vi "Version_4.9_8_on-chip_valves_for25ulSyringe_withModfied_Plunging.vi"() -> ()   [LabVIEW 2020] (continued)
                            n7037 = call "PortChanger (SubVI).vi"("Port Number"=w7491, "VISA Refnum in"=w7492) -> ()  [unwired: 10 in]
                          }
                          frame #1 {
                            n7038 = local read "VISA Refnum in\nfor Pump"() -> (w7493:refnum<visa-resource-name>)
                            n7039 = call "ProcessCompletionWaiter (SubVI).vi"("VISA Refnum in"=w7493) -> ()  [unwired: 11 in]
                          }
                          frame #2 {
                            n7040 = local read "Buffer-A2 PickUp \nFlow Rate (ul/min)"() -> (w7496:dbl)
                            n7041 = local read "Buffer-A2 Pumping\nResolution"() -> (w7495:T2)
                            n7042 = local read "VISA Refnum in\nfor Pump"() -> (w7498:refnum<visa-resource-name>)
                            n7043 = local read "Reminder of the \nVolume to be \nPumped"() -> (w7494:dbl)
                            n7044 = local read "Volume of Syringe"() -> (w7497:dbl)
                            n7045 = call "RPickUp(SubVI).vi"("Volume to be picked up"=w7494, "Volume of Syringe"=w7497, "Resolution of PickUP"=w7495, "PickUp Flow Rate (ul/min)"=w7496, "VISA Refnum in"=w7498) -> ()  [unwired: 6 in, 1 out]
                          }
                          frame #3 {
                            n7046 = local read "Stopper that ends \nthe main loops"() -> (w7499:bool)
                            n7047 = local read "VISA Refnum in\nfor Pump"() -> (w7500:refnum<visa-resource-name>)
                            n7048 = case shown="True" w7499 {
                              frame False {
                              }
                              frame True {
                                n7049 = local read "VISA Refnum in\nfor Pump"() -> (w7501:refnum<visa-resource-name>)
                                n7050 = call "HardStopCurrentProcess (SubVI).vi"("VISA Refnum in"=w7501) -> ()  [unwired: 11 in]
                              }
                            }
                            n7051 = call "ProcessCompletionWaiter (SubVI).vi"("VISA Refnum in"=w7500) -> ()  [unwired: 11 in]
                          }
                          frame #4 {
                            # "Reads the initial Plunger Position for computing the volume dispensed"
                            n7052 = local read "VISA Refnum in\nfor Pump"() -> (w7503:refnum<visa-resource-name>)
                            n7053 = call "AbsolutePlungerPosition (SubVI).vi"("VISA Refnum in"=w7503) -> ("Plunger Position"=w7502:i32)  [unwired: 10 in]
                            n7054 = local write "Initial Plunger Position"(w7502) -> ()
                          }
                          frame #5 {
                            # "Switch to Port-2"
                            # "Port-2 of the pump is conncted to column-1 of chip"
                            n7055 = local read "VISA Refnum in\nfor Pump"() -> (w7505:refnum<visa-resource-name>)
                            n7056 = call "PortChanger (SubVI).vi"("Port Number"="2", "VISA Refnum in"=w7505) -> ()  [unwired: 10 in]
                          }
                          frame #6 {
                            n7057 = local read "Stopper that ends \nthe main loops"() -> (w7506:bool)
                            n7058 = local read "VISA Refnum in\nfor Pump"() -> (w7507:refnum<visa-resource-name>)
                            n7059 = case shown="True" w7506 {
                              frame False {
                              }
                              frame True {
                                n7060 = local read "VISA Refnum in\nfor Pump"() -> (w7508:refnum<visa-resource-name>)
                                n7061 = call "HardStopCurrentProcess (SubVI).vi"("VISA Refnum in"=w7508) -> ()  [unwired: 11 in]
                              }
                            }
                            n7062 = call "ProcessCompletionWaiter (SubVI).vi"("VISA Refnum in"=w7507) -> ()  [unwired: 11 in]
                          }
                          frame #7 {
                            # "Keeps the AMF valve after column-1 open and valve after column-2 closed"
                            n7063 = local read "Buffer-A2 Dispense\nFlow Rate (ul/min)"() -> (w7521:dbl)
                            n7064 = local read "Buffer-A2 Pumping\nResolution"() -> (w7520:T2)
                            n7065 = local read "VISA Refnum in\nfor Pump"() -> (w7523:refnum<visa-resource-name>)
                            n7066 = local write "Pause Data Collection"(FALSE ("Pause Data Collection")) -> ()
                            n7067 = local write "Valve V3 Open"(FALSE ("Valve V3 Open")) -> ()
                            n7068 = local write "Valve V4 Open"(FALSE ("Valve V4 Open")) -> ()
                            n7069 = local write "Valve V1 Open"(TRUE ("Valve V1 Open")) -> ()
                            n7070 = local write "Valve V2 Open"(TRUE ("Valve V2 Open")) -> ()
                            n7071 = local read "Volume of Syringe"() -> (w7522:dbl)
                            n7072 = call "GoToAbsolutePosition(SubVI).vi"("Absolute Volume Position in Syringe (in ul)"=0.0 ("Volume to be Dispensed"), "Volume of Syringe"=w7522, "Resolution of Pumping"=w7520, "Flow Rate (ul/min)"=w7521, "VISA Refnum in"=w7523) -> ()  [unwired: 6 in, 1 out]
                            n7073 = local write "External Valve \nOpen"(TRUE ("External Valve \nOpen")) -> ()
                            n7074 = local write "Valve V5 Open"(FALSE ("Valve V5 Open")) -> ()
                            n7075 = local write "Valve V8 Open"(FALSE ("Valve V8 Open")) -> ()
                            n7076 = local write "Valve V6 Open"(FALSE ("Valve V6 Open")) -> ()
                            n7077 = local write "Valve V7 Open"(FALSE ("Valve V7 Open")) -> ()
                          }
                          frame #8 {
                            n7078 = local read "Initial Plunger Position"() -> (w7526:dbl)
                            n7079 = local read "Buffer-A2 Pumping\nResolution"() -> (w7525:T2)
                            n7080 = local read "VISA Refnum in\nfor Pump"() -> (w7527:refnum<visa-resource-name>)
                            n7081 = local read "Volume of Syringe"() -> (w7524:dbl)
                            n7082 = while {
                              tunnel: w7526 -> [w7533]
                              tunnel: w7527 -> [w7532]
                              tunnel: w7525 -> [w7531]
                              tunnel: w7524 -> [w7530]
                              stop <- w7528 stop-if-true
                              n7083 = Wait (ms)(milliseconds to wait=u32 100) -> ()  [unwired: 1 out]
                              n7084 = stacked-sequence {
                                tunnel: w7533 -> [w7539 _]
                                tunnel: w7532 -> [w7538 w7559]
                                tunnel: w7531 -> [w7537 _]
                                tunnel: w7530 -> [w7536 _]
                                tunnel: [_ w7556] -> w7528
                                frame #0 {
                                n7085 = call "AbsolutePlungerPosition (SubVI).vi"("VISA Refnum in"=w7538) -> ("Plunger Position"=w7535:i32)  [unwired: 10 in]
                                n7086 = case shown="\"Standard Pumping\", Default" w7537 {
                                tunnel: w7539 -> [w7544 w7553]
                                tunnel: w7535 -> [w7545 w7552]
                                tunnel: [w7543 w7550] -> w7534
                                tunnel: w7536 -> [w7542 w7551]
                                frame "Standard Pumping", Default {
                                n7087 = Subtract(x=w7544, y=w7545) -> (x-y=w7541:dbl)
                                n7088 = Absolute Value(x=w7541) -> (abs(x)=w7540:dbl)
                                n7089 = Multiply(x=w7540, y=w7542) -> (x*y=w7547:dbl)
                                n7090 = Divide(x=w7547, y=3000.0) -> (x/y=w7543:dbl)
                                }
                                frame "High Resolution Pumping" {
                                n7091 = Subtract(x=w7553, y=w7552) -> (x-y=w7549:dbl)
                                n7092 = Absolute Value(x=w7549) -> (abs(x)=w7548:dbl)
                                n7093 = Multiply(x=w7548, y=w7551) -> (x*y=w7555:dbl)
                                n7094 = Divide(x=w7555, y=24000.0) -> (x/y=w7550:dbl)
                                }
                                }
                                n7095 = local write "Volume being Injected \nin this process"(w7534) -> ()
                                }
                                frame #1 {
                                n7096 = local read "Stop for End of \nExperiment \nand Data Writing"() -> (w7558:bool)
                                n7097 = call "LSPOneStatus (SubVI).vi"("VISA Refnum in"=w7559) -> ("read buffer"=w7561:string)  [unwired: 10 in]
                                n7098 = call <vilib>:"Trim Whitespace.vi"("string"=w7561) -> ("trimmed string"=w7560:string)  [unwired: 1 in]
                                n7099 = Equal?(x=w7560, y="/0`\u0003") -> (x = y?=w7557:bool)
                                n7100 = Or(x=w7557, y=w7558) -> (x .or. y?=w7556:bool)
                                }
                              }
                            }
                          }
                          frame #9 {
                            n7101 = local read "Stop for End of \nExperiment \nand Data Writing"() -> (w7563:bool)
                            n7102 = local write "Pause Data Collection"(TRUE ("Pause Data Collection")) -> ()
                            n7103 = local write "Valve V3 Open"(FALSE ("Valve V3 Open")) -> ()
                            n7104 = local write "Valve V2 Open"(FALSE ("Valve V2 Open")) -> ()
                            n7105 = local write "Valve V4 Open"(FALSE ("Valve V4 Open")) -> ()
                            n7106 = local write "Start the Process"(FALSE) -> ()
                            n7107 = local write "Valve V1 Open"(FALSE ("Valve V1 Open")) -> ()
                            n7108 = case shown="True" w7563 {
                              frame False {
                              }
                              frame True {
                                n7109 = local read "VISA Refnum in\nfor Pump"() -> (w7574:refnum<visa-resource-name>)
                                n7110 = call "HardStopCurrentProcess (SubVI).vi"("VISA Refnum in"=w7574) -> ()  [unwired: 11 in]
                              }
                            }
                            n7111 = Wait (ms)(milliseconds to wait=u32 500) -> ()  [unwired: 1 out]
                            n7112 = local write "Valve V5 Open"(FALSE ("Valve V5 Open")) -> ()
                            n7113 = local write "Valve V6 Open"(FALSE ("Valve V6 Open")) -> ()
                            n7114 = local write "Valve V7 Open"(FALSE ("Valve V7 Open")) -> ()
                          }
                          frame #10 {
                            n7115 = local write "Volume being Injected \nin this process"(0.0 ("Volume being Injected \nin this process")) -> ()
                          }
                        }
                      }
                    }
                  }
                }
              }
              frame True {
                n7116 = local write "Pause Data Collection"(FALSE ("Pause Data Collection")) -> ()
              }
            }
          }
          frame "Inject Buffer B, Column 1 with 4 SOD Valves" {
            n7117 = local read "Stopper that ends \nthe main loops"() -> (w7577:bool)
            n7118 = case shown="False" w7577 {
              frame False {
                n7119 = local read "Start the Process"() -> (w7578:bool)
                n7120 = case shown="True" w7578 {
                  frame False {
                    n7121 = local read "Stopper that ends \nthe main loops"() -> (w7580:bool)
                    n7122 = local read "Start the Process"() -> (w7579:bool)
                    n7123 = Or(x=w7580, y=w7579) -> (x .or. y?=w7581:bool)
                    n7124 = case shown="False" w7581 {
                      frame False {
                        n7125 = while {
                          stop <- w7584 stop-if-true
                          n7126 = local read "Stop for End of \nExperiment \nand Data Writing"() -> (w7583:bool)
                          n7127 = local read "Stopper that ends \nthe main loops"() -> (w7586:bool)
                          n7128 = local read "Start the Process"() -> (w7585:bool)
                          n7129 = Wait (ms)(milliseconds to wait=u32 10) -> ()  [unwired: 1 out]
                          n7130 = Or(x=w7586, y=w7585) -> (x .or. y?=w7584:bool)
                          n7131 = local write "Stopper that ends \nthe main loops"(w7583) -> ()
                        }
                        n7132 = One Button Dialog(message="Please Select the Process and Press 'Start the Process' Button") -> ()  [unwired: 1 in, 1 out]
                      }
                      frame True {
                      }
                    }
                  }
                  frame True {
                    n7133 = stacked-sequence {
                      frame #0 {
                        n7134 = local read "Apparent Volume\nof Syringe"() -> (w7590:dbl)
                        n7135 = local read "Buffer-B Volume \nto be  Pumped"() -> (w7591:dbl)
                        n7136 = Quotient & Remainder(x=w7591, y=w7590) -> (x-y*floor(x/y)=w7588:dbl, floor(x/y)=w7589:dbl)
                        n7137 = for {
                          N: w7589 -> [_]
                          n7138 = stacked-sequence {
                            frame #0 {
                              # "Switch to Port-7"
                              # "Port-7 of pump is connected to Buffer-B"
                              n7139 = local read "VISA Refnum in\nfor Pump"() -> (w7593:refnum<visa-resource-name>)
                              n7140 = local read "Port for \nB-Elution"() -> (w7592:string)
                              n7141 = call "PortChanger (SubVI).vi"("Port Number"=w7592, "VISA Refnum in"=w7593) -> ()  [unwired: 10 in]
                            }
                            frame #1 {
                              n7142 = local read "VISA Refnum in\nfor Pump"() -> (w7594:refnum<visa-resource-name>)
                              n7143 = call "ProcessCompletionWaiter (SubVI).vi"("VISA Refnum in"=w7594) -> ()  [unwired: 11 in]
                            }
                            frame #2 {
                              n7144 = local read "Buffer-B PickUp \nFlow Rate (ul/min)"() -> (w7597:dbl)
                              n7145 = local read "Buffer-B Pumping\nResolution"() -> (w7596:T2)
                              n7146 = local read "VISA Refnum in\nfor Pump"() -> (w7599:refnum<visa-resource-name>)
                              n7147 = local read "Apparent Volume\nof Syringe"() -> (w7595:dbl)
                              n7148 = local read "Volume of Syringe"() -> (w7598:dbl)
                              n7149 = call "RPickUp(SubVI).vi"("Volume to be picked up"=w7595, "Volume of Syringe"=w7598, "Resolution of PickUP"=w7596, "PickUp Flow Rate (ul/min)"=w7597, "VISA Refnum in"=w7599) -> ()  [unwired: 6 in, 1 out]
                            }
                            frame #3 {
                              n7150 = local read "Stopper that ends \nthe main loops"() -> (w7600:bool)
                              n7151 = local read "VISA Refnum in\nfor Pump"() -> (w7601:refnum<visa-resource-name>)
                              n7152 = case shown="True" w7600 {
                                frame False {
                                }
                                frame True {
                                n7153 = local read "VISA Refnum in\nfor Pump"() -> (w7602:refnum<visa-resource-name>)
                                n7154 = call "HardStopCurrentProcess (SubVI).vi"("VISA Refnum in"=w7602) -> ()  [unwired: 11 in]
                                }
                              }
                              n7155 = call "ProcessCompletionWaiter (SubVI).vi"("VISA Refnum in"=w7601) -> ()  [unwired: 11 in]
                            }
                            frame #4 {
                              # "Reads the initial Plunger Position for computing the volume dispensed"
                              n7156 = local read "VISA Refnum in\nfor Pump"() -> (w7604:refnum<visa-resource-name>)
                              n7157 = call "AbsolutePlungerPosition (SubVI).vi"("VISA Refnum in"=w7604) -> ("Plunger Position"=w7603:i32)  [unwired: 10 in]
                              n7158 = local write "Initial Plunger Position"(w7603) -> ()
                            }
                            frame #5 {
                              # "Switch to Port-8"
                              # "Port-8 of the pump is conncted to column-1 of chip"
                              n7159 = local read "VISA Refnum in\nfor Pump"() -> (w7606:refnum<visa-resource-name>)
                              n7160 = call "PortChanger (SubVI).vi"("Port Number"="8", "VISA Refnum in"=w7606) -> ()  [unwired: 10 in]
                            }
                            frame #6 {
                              n7161 = local read "Stopper that ends \nthe main loops"() -> (w7607:bool)
                              n7162 = local read "VISA Refnum in\nfor Pump"() -> (w7608:refnum<visa-resource-name>)
                              n7163 = case shown="True" w7607 {
                                frame False {
                                }
                                frame True {
                                n7164 = local read "VISA Refnum in\nfor Pump"() -> (w7609:refnum<visa-resource-name>)
                                n7165 = call "HardStopCurrentProcess (SubVI).vi"("VISA Refnum in"=w7609) -> ()  [unwired: 11 in]
                                }
                              }
                              n7166 = call "ProcessCompletionWaiter (SubVI).vi"("VISA Refnum in"=w7608) -> ()  [unwired: 11 in]
                            }
                            frame #7 {
                              # "Keeps the AMF valve after column-1 open and valve after column-2 closed"
                              n7167 = local read "Buffer-B Dispense\nFlow Rate (ul/min)"() -> (w7622:dbl)
                              n7168 = local read "Buffer-B Pumping\nResolution"() -> (w7621:T2)
                              n7169 = local read "VISA Refnum in\nfor Pump"() -> (w7624:refnum<visa-resource-name>)
                              n7170 = local write "Pause Data Collection"(FALSE ("Pause Data Collection")) -> ()
                              n7171 = local write "Valve V1 Open"(TRUE ("Valve V1 Open")) -> ()
                              n7172 = local write "Valve V3 Open"(FALSE ("Valve V3 Open")) -> ()
                              n7173 = local write "Valve V2 Open"(TRUE ("Valve V2 Open")) -> ()
                              n7174 = local write "Valve V4 Open"(FALSE ("Valve V4 Open")) -> ()
                              n7175 = local read "Volume of Syringe"() -> (w7623:dbl)
                              n7176 = call "GoToAbsolutePosition(SubVI).vi"("Absolute Volume Position in Syringe (in ul)"=0.0 ("Volume to be Dispensed"), "Volume of Syringe"=w7623, "Resolution of Pumping"=w7621, "Flow Rate (ul/min)"=w7622, "VISA Refnum in"=w7624) -> ()  [unwired: 6 in, 1 out]
                              n7177 = local write "External Valve \nOpen"(TRUE ("External Valve \nOpen")) -> ()
                              n7178 = local write "Valve V8 Open"(FALSE ("Valve V8 Open")) -> ()
                              n7179 = local write "Valve V6 Open"(FALSE ("Valve V6 Open")) -> ()
                              n7180 = local write "Valve V7 Open"(FALSE ("Valve V7 Open")) -> ()
                              n7181 = local write "Valve V5 Open"(FALSE ("Valve V5 Open")) -> ()
                            }
                            frame #8 {
                              n7182 = local read "Initial Plunger Position"() -> (w7627:dbl)
                              n7183 = local read "Buffer-B Pumping\nResolution"() -> (w7626:T2)
                              n7184 = local read "VISA Refnum in\nfor Pump"() -> (w7628:refnum<visa-resource-name>)
                              n7185 = local read "Volume of Syringe"() -> (w7625:dbl)
                              n7186 = while {
                                tunnel: w7627 -> [w7634]
                                tunnel: w7628 -> [w7633]
                                tunnel: w7626 -> [w7632]
                                tunnel: w7625 -> [w7631]
                                stop <- w7629 stop-if-true
                                n7187 = Wait (ms)(milliseconds to wait=u32 100) -> ()  [unwired: 1 out]
                                n7188 = stacked-sequence {
                                tunnel: w7634 -> [w7640 _]
                                tunnel: w7633 -> [w7639 w7660]
                                tunnel: w7632 -> [w7638 _]
                                tunnel: w7631 -> [w7637 _]
                                tunnel: [_ w7657] -> w7629
                                frame #0 {
                                n7189 = call "AbsolutePlungerPosition (SubVI).vi"("VISA Refnum in"=w7639) -> ("Plunger Position"=w7636:i32)  [unwired: 10 in]
                                n7190 = case shown="\"Standard Pumping\", Default" w7638 {
                                tunnel: w7640 -> [w7645 w7654]
                                tunnel: w7636 -> [w7646 w7653]
                                tunnel: [w7644 w7651] -> w7635
                                tunnel: w7637 -> [w7643 w7652]
                                frame "Standard Pumping", Default {
                                n7191 = Subtract(x=w7645, y=w7646) -> (x-y=w7642:dbl)
                                n7192 = Absolute Value(x=w7642) -> (abs(x)=w7641:dbl)
                                n7193 = Multiply(x=w7641, y=w7643) -> (x*y=w7648:dbl)
                                n7194 = Divide(x=w7648, y=3000.0) -> (x/y=w7644:dbl)
                                }
                                frame "High Resolution Pumping" {
                                n7195 = Subtract(x=w7654, y=w7653) -> (x-y=w7650:dbl)
                                n7196 = Absolute Value(x=w7650) -> (abs(x)=w7649:dbl)
                                n7197 = Multiply(x=w7649, y=w7652) -> (x*y=w7656:dbl)
                                n7198 = Divide(x=w7656, y=24000.0) -> (x/y=w7651:dbl)
                                }
                                }
                                n7199 = local write "Volume being Injected \nin this process"(w7635) -> ()
                                }
                                frame #1 {
                                n7200 = call "LSPOneStatus (SubVI).vi"("VISA Refnum in"=w7660) -> ("read buffer"=w7662:string)  [unwired: 10 in]
                                n7201 = local read "Stopper that ends \nthe main loops"() -> (w7659:bool)
                                n7202 = call <vilib>:"Trim Whitespace.vi"("string"=w7662) -> ("trimmed string"=w7661:string)  [unwired: 1 in]
                                n7203 = Equal?(x=w7661, y="/0`\u0003") -> (x = y?=w7658:bool)
                                n7204 = Or(x=w7658, y=w7659) -> (x .or. y?=w7657:bool)
                                }
                                }
                              }
                            }
                            frame #9 {
                              n7205 = local read "Stopper that ends \nthe main loops"() -> (w7664:bool)
                              n7206 = local write "Pause Data Collection"(TRUE ("Pause Data Collection")) -> ()
                              n7207 = local write "Valve V2 Open"(FALSE ("Valve V2 Open")) -> ()
                              n7208 = local write "Valve V4 Open"(FALSE ("Valve V4 Open")) -> ()
                              n7209 = Wait (ms)(milliseconds to wait=u32 500) -> ()  [unwired: 1 out]
                              n7210 = local write "Valve V1 Open"(FALSE ("Valve V1 Open")) -> ()
                              n7211 = local write "Valve V3 Open"(FALSE ("Valve V3 Open")) -> ()
                              n7212 = case shown="True" w7664 {
                                frame False {
                                }
                                frame True {
                                n7213 = local read "VISA Refnum in\nfor Pump"() -> (w7674:refnum<visa-resource-name>)
                                n7214 = call "HardStopCurrentProcess (SubVI).vi"("VISA Refnum in"=w7674) -> ()  [unwired: 11 in]
                                }
                              }
                              n7215 = local write "Valve V5 Open"(FALSE ("Valve V5 Open")) -> ()
                              n7216 = local write "Valve V6 Open"(FALSE ("Valve V6 Open")) -> ()
                              n7217 = local write "Valve V7 Open"(FALSE ("Valve V7 Open")) -> ()
                            }
                            frame #10 {
                              n7218 = local write "Volume being Injected \nin this process"(0.0 ("Volume being Injected \nin this process")) -> ()
                            }
                          }
                        }
                        n7219 = local write "Reminder of the \nVolume to be \nPumped"(w7588) -> ()
                      }
                      frame #1 {
                        n7220 = stacked-sequence {
                          frame #0 {
                            # "Switch to Port-7"
                            # "Port-7 of pump is connected to Buffer-B"
                            n7221 = local read "VISA Refnum in\nfor Pump"() -> (w7677:refnum<visa-resource-name>)
                            n7222 = local read "Port for \nB-Elution"() -> (w7676:string)
                            n7223 = call "PortChanger (SubVI).vi"("Port Number"=w7676, "VISA Refnum in"=w7677) -> ()  [unwired: 10 in]
                          }
                          frame #1 {
                            n7224 = local read "VISA Refnum in\nfor Pump"() -> (w7678:refnum<visa-resource-name>)
                            n7225 = call "ProcessCompletionWaiter (SubVI).vi"("VISA Refnum in"=w7678) -> ()  [unwired: 11 in]
                          }
                          frame #2 {
                            n7226 = local read "Buffer-B PickUp \nFlow Rate (ul/min)"() -> (w7681:dbl)
                            n7227 = local read "Buffer-B Pumping\nResolution"() -> (w7680:T2)
                            n7228 = local read "VISA Refnum in\nfor Pump"() -> (w7683:refnum<visa-resource-name>)
                            n7229 = local read "Reminder of the \nVolume to be \nPumped"() -> (w7679:dbl)
                            n7230 = local read "Volume of Syringe"() -> (w7682:dbl)
                            n7231 = call "RPickUp(SubVI).vi"("Volume to be picked up"=w7679, "Volume of Syringe"=w7682, "Resolution of PickUP"=w7680, "PickUp Flow Rate (ul/min)"=w7681, "VISA Refnum in"=w7683) -> ()  [unwired: 6 in, 1 out]
                          }
                          frame #3 {
                            n7232 = local read "Stopper that ends \nthe main loops"() -> (w7684:bool)
                            n7233 = local read "VISA Refnum in\nfor Pump"() -> (w7685:refnum<visa-resource-name>)
                            n7234 = case shown="True" w7684 {
                              frame False {
                              }
                              frame True {
                                n7235 = local read "VISA Refnum in\nfor Pump"() -> (w7686:refnum<visa-resource-name>)
                                n7236 = call "HardStopCurrentProcess (SubVI).vi"("VISA Refnum in"=w7686) -> ()  [unwired: 11 in]
                              }
                            }
                            n7237 = call "ProcessCompletionWaiter (SubVI).vi"("VISA Refnum in"=w7685) -> ()  [unwired: 11 in]
                          }
                          frame #4 {
                            # "Reads the initial Plunger Position for computing the volume dispensed"
                            n7238 = local read "VISA Refnum in\nfor Pump"() -> (w7688:refnum<visa-resource-name>)
                            n7239 = call "AbsolutePlungerPosition (SubVI).vi"("VISA Refnum in"=w7688) -> ("Plunger Position"=w7687:i32)  [unwired: 10 in]
                            n7240 = local write "Initial Plunger Position"(w7687) -> ()
                          }
                          frame #5 {
                            # "Switch to Port-2"
                            # "Port-2 of the pump is conncted to column-1 of chip"
                            n7241 = local read "VISA Refnum in\nfor Pump"() -> (w7690:refnum<visa-resource-name>)
                            n7242 = call "PortChanger (SubVI).vi"("Port Number"="8", "VISA Refnum in"=w7690) -> ()  [unwired: 10 in]
                          }
                          frame #6 {
                            n7243 = local read "Stopper that ends \nthe main loops"() -> (w7691:bool)
                            n7244 = local read "VISA Refnum in\nfor Pump"() -> (w7692:refnum<visa-resource-name>)
                            n7245 = case shown="True" w7691 {
                              frame False {
                              }
                              frame True {
                                n7246 = local read "VISA Refnum in\nfor Pump"() -> (w7693:refnum<visa-resource-name>)
                                n7247 = call "HardStopCurrentProcess (SubVI).vi"("VISA Refnum in"=w7693) -> ()  [unwired: 11 in]
                              }
                            }
                            n7248 = call "ProcessCompletionWaiter (SubVI).vi"("VISA Refnum in"=w7692) -> ()  [unwired: 11 in]
                          }
                          frame #7 {
                            # "Keeps the AMF valve after column-1 open and valve after column-2 closed"
                            n7249 = local read "Buffer-B Dispense\nFlow Rate (ul/min)"() -> (w7706:dbl)
                            n7250 = local read "Buffer-B Pumping\nResolution"() -> (w7705:T2)
                            n7251 = local read "VISA Refnum in\nfor Pump"() -> (w7708:refnum<visa-resource-name>)
                            n7252 = local write "Pause Data Collection"(FALSE ("Pause Data Collection")) -> ()
                            n7253 = local write "Valve V1 Open"(TRUE ("Valve V1 Open")) -> ()
                            n7254 = local write "Valve V3 Open"(FALSE ("Valve V3 Open")) -> ()
                            n7255 = local write "Valve V2 Open"(TRUE ("Valve V2 Open")) -> ()
                            n7256 = local write "Valve V4 Open"(FALSE ("Valve V4 Open")) -> ()
                            n7257 = local read "Volume of Syringe"() -> (w7707:dbl)
                            n7258 = call "GoToAbsolutePosition(SubVI).vi"("Absolute Volume Position in Syringe (in ul)"=0.0 ("Volume to be Dispensed"), "Volume of Syringe"=w7707, "Resolution of Pumping"=w7705, "Flow Rate (ul/min)"=w7706, "VISA Refnum in"=w7708) -> ()  [unwired: 6 in, 1 out]
                            n7259 = local write "External Valve \nOpen"(TRUE ("External Valve \nOpen")) -> ()
                            n7260 = local write "Valve V8 Open"(FALSE ("Valve V8 Open")) -> ()
                            n7261 = local write "Valve V6 Open"(FALSE ("Valve V6 Open")) -> ()
                            n7262 = local write "Valve V7 Open"(FALSE ("Valve V7 Open")) -> ()
                            n7263 = local write "Valve V5 Open"(FALSE ("Valve V5 Open")) -> ()
                          }
                          frame #8 {
                            n7264 = local read "Initial Plunger Position"() -> (w7711:dbl)
                            n7265 = local read "Buffer-B Pumping\nResolution"() -> (w7710:T2)
                            n7266 = local read "VISA Refnum in\nfor Pump"() -> (w7712:refnum<visa-resource-name>)
                            n7267 = local read "Volume of Syringe"() -> (w7709:dbl)
                            n7268 = while {
                              tunnel: w7711 -> [w7718]
                              tunnel: w7712 -> [w7717]
                              tunnel: w7710 -> [w7716]
                              tunnel: w7709 -> [w7715]
                              stop <- w7713 stop-if-true
                              n7269 = Wait (ms)(milliseconds to wait=u32 100) -> ()  [unwired: 1 out]
                              n7270 = stacked-sequence {
                                tunnel: w7718 -> [w7724 _]
                                tunnel: w7717 -> [w7723 w7744]
                                tunnel: w7716 -> [w7722 _]
                                tunnel: w7715 -> [w7721 _]
                                tunnel: [_ w7741] -> w7713
                                frame #0 {
                                n7271 = call "AbsolutePlungerPosition (SubVI).vi"("VISA Refnum in"=w7723) -> ("Plunger Position"=w7720:i32)  [unwired: 10 in]
                                n7272 = case shown="\"Standard Pumping\", Default" w7722 {
                                tunnel: w7724 -> [w7729 w7738]
                                tunnel: w7720 -> [w7730 w7737]
                                tunnel: [w7728 w7735] -> w7719
                                tunnel: w7721 -> [w7727 w7736]
                                frame "Standard Pumping", Default {
                                n7273 = Subtract(x=w7729, y=w7730) -> (x-y=w7726:dbl)
                                n7274 = Absolute Value(x=w7726) -> (abs(x)=w7725:dbl)
                                n7275 = Multiply(x=w7725, y=w7727) -> (x*y=w7732:dbl)
                                n7276 = Divide(x=w7732, y=3000.0) -> (x/y=w7728:dbl)
                                }
                                frame "High Resolution Pumping" {
                                n7277 = Subtract(x=w7738, y=w7737) -> (x-y=w7734:dbl)
                                n7278 = Absolute Value(x=w7734) -> (abs(x)=w7733:dbl)
                                n7279 = Multiply(x=w7733, y=w7736) -> (x*y=w7740:dbl)
                                n7280 = Divide(x=w7740, y=24000.0) -> (x/y=w7735:dbl)
                                }
                                }
                                n7281 = local write "Volume being Injected \nin this process"(w7719) -> ()
                                }
                                frame #1 {
                                n7282 = call "LSPOneStatus (SubVI).vi"("VISA Refnum in"=w7744) -> ("read buffer"=w7746:string)  [unwired: 10 in]
                                n7283 = local read "Stopper that ends \nthe main loops"() -> (w7743:bool)
                                n7284 = call <vilib>:"Trim Whitespace.vi"("string"=w7746) -> ("trimmed string"=w7745:string)  [unwired: 1 in]
                                n7285 = Equal?(x=w7745, y="/0`\u0003") -> (x = y?=w7742:bool)
                                n7286 = Or(x=w7742, y=w7743) -> (x .or. y?=w7741:bool)
                                }
                              }
                            }
                          }
                          frame #9 {
                            n7287 = local read "Stopper that ends \nthe main loops"() -> (w7748:bool)
                            n7288 = local write "Pause Data Collection"(TRUE ("Pause Data Collection")) -> ()
                            n7289 = local write "Valve V2 Open"(FALSE ("Valve V2 Open")) -> ()
                            n7290 = local write "Start the Process"(FALSE) -> ()
                            n7291 = local write "Valve V4 Open"(FALSE ("Valve V4 Open")) -> ()
                            n7292 = Wait (ms)(milliseconds to wait=u32 500) -> ()  [unwired: 1 out]
                            n7293 = local write "Valve V1 Open"(FALSE ("Valve V1 Open")) -> ()
                            n7294 = local write "Valve V3 Open"(FALSE ("Valve V3 Open")) -> ()
                            n7295 = case shown="True" w7748 {
                              frame False {
                              }
                              frame True {
                                n7296 = local read "VISA Refnum in\nfor Pump"() -> (w7759:refnum<visa-resource-name>)
                                n7297 = call "HardStopCurrentProcess (SubVI).vi"("VISA Refnum in"=w7759) -> ()  [unwired: 11 in]
                              }
                            }
                            n7298 = local write "Valve V5 Open"(FALSE ("Valve V5 Open")) -> ()
                            n7299 = local write "Valve V6 Open"(FALSE ("Valve V6 Open")) -> ()
                            n7300 = local write "Valve V7 Open"(FALSE ("Valve V7 Open")) -> ()
                          }
                          frame #10 {
                            n7301 = local write "Volume being Injected \nin this process"(0.0 ("Volume being Injected \nin this process")) -> ()
                          }
                        }
                      }
                    }
                  }
                }
              }
              frame True {
                n7302 = local write "Pause Data Collection"(FALSE ("Pause Data Collection")) -> ()
              }
            }
          }
          frame "Inject Buffer C2, Column 2 with 4 SOD Valves" {
            n7303 = local read "Stopper that ends \nthe main loops"() -> (w7762:bool)
            n7304 = case shown="False" w7762 {
              frame False {
                n7305 = local read "Start the Process"() -> (w7763:bool)
                n7306 = case shown="True" w7763 {
                  frame False {
                    n7307 = local read "Stopper that ends \nthe main loops"() -> (w7765:bool)
                    n7308 = local read "Start the Process"() -> (w7764:bool)
                    n7309 = Or(x=w7765, y=w7764) -> (x .or. y?=w7766:bool)
                    n7310 = case shown="False" w7766 {
                      frame False {
                        n7311 = while {
                          stop <- w7769 stop-if-true
                          n7312 = local read "Stop for End of \nExperiment \nand Data Writing"() -> (w7768:bool)
                          n7313 = local read "Stopper that ends \nthe main loops"() -> (w7771:bool)
                          n7314 = local read "Start the Process"() -> (w7770:bool)
                          n7315 = Wait (ms)(milliseconds to wait=u32 10) -> ()  [unwired: 1 out]
                          n7316 = Or(x=w7771, y=w7770) -> (x .or. y?=w7769:bool)
                          n7317 = local write "Stopper that ends \nthe main loops"(w7768) -> ()
                        }
                        n7318 = One Button Dialog(message="Please Select the Process and Press 'Start the Process' Button") -> ()  [unwired: 1 in, 1 out]
                      }
                      frame True {
                      }
                    }
                  }
                  frame True {
                    n7319 = stacked-sequence {
                      frame #0 {
                        n7320 = local read "Apparent Volume\nof Syringe"() -> (w7775:dbl)
                        n7321 = local read "Buffer-C2 Volume \nto be Pumped"() -> (w7776:dbl)
                        n7322 = Quotient & Remainder(x=w7776, y=w7775) -> (x-y*floor(x/y)=w7773:dbl, floor(x/y)=w7774:dbl)
                        n7323 = for {
                          N: w7774 -> [_]
                          n7324 = stacked-sequence {
                            frame #0 {
                              # "Switch to Port-5/8"
                              # "Port-5/8 of pump is connected to Buffer-C/Buffer-A"
                              n7325 = local read "VISA Refnum in\nfor Pump"() -> (w7778:refnum<visa-resource-name>)
                              n7326 = local read "Port for \nC2-Elution"() -> (w7777:string)
                              n7327 = call "PortChanger (SubVI).vi"("Port Number"=w7777, "VISA Refnum in"=w7778) -> ()  [unwired: 10 in]
                            }
                            frame #1 {
                              n7328 = local read "VISA Refnum in\nfor Pump"() -> (w7779:refnum<visa-resource-name>)
                              n7329 = call "ProcessCompletionWaiter (SubVI).vi"("VISA Refnum in"=w7779) -> ()  [unwired: 11 in]
                            }
                            frame #2 {
                              n7330 = local read "Buffer-C2 PickUp \nFlow Rate (ul/min)"() -> (w7782:dbl)
                              n7331 = local read "Buffer-C2 Pumping\nResolution"() -> (w7781:T2)
                              n7332 = local read "VISA Refnum in\nfor Pump"() -> (w7784:refnum<visa-resource-name>)
                              n7333 = local read "Apparent Volume\nof Syringe"() -> (w7780:dbl)
                              n7334 = local read "Volume of Syringe"() -> (w7783:dbl)
                              n7335 = call "RPickUp(SubVI).vi"("Volume to be picked up"=w7780, "Volume of Syringe"=w7783, "Resolution of PickUP"=w7781, "PickUp Flow Rate (ul/min)"=w7782, "VISA Refnum in"=w7784) -> ()  [unwired: 6 in, 1 out]
                            }
                            frame #3 {
                              n7336 = local read "Stopper that ends \nthe main loops"() -> (w7785:bool)
                              n7337 = local read "VISA Refnum in\nfor Pump"() -> (w7786:refnum<visa-resource-name>)
                              n7338 = case shown="True" w7785 {
                                frame False {
                                }
                                frame True {
                                n7339 = local read "VISA Refnum in\nfor Pump"() -> (w7787:refnum<visa-resource-name>)
                                n7340 = call "HardStopCurrentProcess (SubVI).vi"("VISA Refnum in"=w7787) -> ()  [unwired: 11 in]
                                }
                              }
                              n7341 = call "ProcessCompletionWaiter (SubVI).vi"("VISA Refnum in"=w7786) -> ()  [unwired: 11 in]
                            }
                            frame #4 {
                              # "Reads the initial Plunger Position for computing the volume dispensed"
                              n7342 = local read "VISA Refnum in\nfor Pump"() -> (w7789:refnum<visa-resource-name>)
                              n7343 = call "AbsolutePlungerPosition (SubVI).vi"("VISA Refnum in"=w7789) -> ("Plunger Position"=w7788:i32)  [unwired: 10 in]
                              n7344 = local write "Initial Plunger Position"(w7788) -> ()
                            }
                            frame #5 {
                              # "Switch to Port-10"
                              # "Port-10 of the pump is conncted to column-2 of chip"
                              n7345 = local read "VISA Refnum in\nfor Pump"() -> (w7791:refnum<visa-resource-name>)
                              n7346 = call "PortChanger (SubVI).vi"("Port Number"="10", "VISA Refnum in"=w7791) -> ()  [unwired: 10 in]
                            }
                            frame #6 {
                              n7347 = local read "Stopper that ends \nthe main loops"() -> (w7792:bool)
                              n7348 = local read "VISA Refnum in\nfor Pump"() -> (w7793:refnum<visa-resource-name>)
                              n7349 = case shown="True" w7792 {
                                frame False {
                                }
                                frame True {
                                n7350 = local read "VISA Refnum in\nfor Pump"() -> (w7794:refnum<visa-resource-name>)
                                n7351 = call "HardStopCurrentProcess (SubVI).vi"("VISA Refnum in"=w7794) -> ()  [unwired: 11 in]
                                }
                              }
                              n7352 = call "ProcessCompletionWaiter (SubVI).vi"("VISA Refnum in"=w7793) -> ()  [unwired: 11 in]
                            }
                            frame #7 {
                              # "Keeps the AMF valve after column-1 closed and valve after column-2 open"
                              n7353 = local read "Buffer-C2 Dispense\nFlow Rate (ul/min)"() -> (w7807:dbl)
                              n7354 = local read "Buffer-C2 Pumping\nResolution"() -> (w7806:T2)
                              n7355 = local read "VISA Refnum in\nfor Pump"() -> (w7809:refnum<visa-resource-name>)
                              n7356 = local write "Pause Data Collection"(FALSE ("Pause Data Collection")) -> ()
                              n7357 = local write "Valve V1 Open"(FALSE ("Valve V1 Open")) -> ()
                              n7358 = local write "Valve V3 Open"(TRUE ("Valve V3 Open")) -> ()
                              n7359 = local write "Valve V2 Open"(FALSE ("Valve V2 Open")) -> ()
                              n7360 = local write "Valve V4 Open"(TRUE ("Valve V4 Open")) -> ()
                              n7361 = local read "Volume of Syringe"() -> (w7808:dbl)
                              n7362 = call "GoToAbsolutePosition(SubVI).vi"("Absolute Volume Position in Syringe (in ul)"=0.0 ("Volume to be Dispensed"), "Volume of Syringe"=w7808, "Resolution of Pumping"=w7806, "Flow Rate (ul/min)"=w7807, "VISA Refnum in"=w7809) -> ()  [unwired: 6 in, 1 out]
                              n7363 = local write "External Valve \nOpen"(FALSE ("External Valve \nOpen")) -> ()
                              n7364 = local write "Valve V8 Open"(FALSE ("Valve V8 Open")) -> ()
                              n7365 = local write "Valve V7 Open"(TRUE ("Valve V7 Open")) -> ()
                              n7366 = local write "Valve V6 Open"(FALSE ("Valve V6 Open")) -> ()
                              n7367 = local write "Valve V5 Open"(TRUE ("Valve V5 Open")) -> ()
                            }
                            frame #8 {
                              n7368 = local read "Initial Plunger Position"() -> (w7812:dbl)
                              n7369 = local read "Buffer-C2 Pumping\nResolution"() -> (w7811:T2)
                              n7370 = local read "VISA Refnum in\nfor Pump"() -> (w7813:refnum<visa-resource-name>)
                              n7371 = local read "Volume of Syringe"() -> (w7810:dbl)
                              n7372 = while {
                                tunnel: w7812 -> [w7819]
                                tunnel: w7813 -> [w7818]
                                tunnel: w7811 -> [w7817]
                                tunnel: w7810 -> [w7816]
                                stop <- w7814 stop-if-true
                                n7373 = Wait (ms)(milliseconds to wait=u32 100) -> ()  [unwired: 1 out]
                                n7374 = stacked-sequence {
                                tunnel: w7819 -> [w7825 _]
                                tunnel: w7818 -> [w7824 w7845]
                                tunnel: w7817 -> [w7823 _]
                                tunnel: w7816 -> [w7822 _]
                                tunnel: [_ w7842] -> w7814
                                frame #0 {
                                n7375 = call "AbsolutePlungerPosition (SubVI).vi"("VISA Refnum in"=w7824) -> ("Plunger Position"=w7821:i32)  [unwired: 10 in]
                                n7376 = case shown="\"Standard Pumping\", Default" w7823 {
                                tunnel: w7825 -> [w7830 w7839]
                                tunnel: w7821 -> [w7831 w7838]
                                tunnel: [w7829 w7836] -> w7820
                                tunnel: w7822 -> [w7828 w7837]
                                frame "Standard Pumping", Default {
                                n7377 = Subtract(x=w7830, y=w7831) -> (x-y=w7827:dbl)
                                n7378 = Absolute Value(x=w7827) -> (abs(x)=w7826:dbl)
                                n7379 = Multiply(x=w7826, y=w7828) -> (x*y=w7833:dbl)
                                n7380 = Divide(x=w7833, y=3000.0) -> (x/y=w7829:dbl)
                                }
                                frame "High Resolution Pumping" {
                                n7381 = Subtract(x=w7839, y=w7838) -> (x-y=w7835:dbl)
                                n7382 = Absolute Value(x=w7835) -> (abs(x)=w7834:dbl)
                                n7383 = Multiply(x=w7834, y=w7837) -> (x*y=w7841:dbl)
                                n7384 = Divide(x=w7841, y=24000.0) -> (x/y=w7836:dbl)
                                }
                                }
                                n7385 = local write "Volume being Injected \nin this process"(w7820) -> ()
                                }
                                frame #1 {
                                n7386 = local read "Stop for End of \nExperiment \nand Data Writing"() -> (w7844:bool)
                                n7387 = call "LSPOneStatus (SubVI).vi"("VISA Refnum in"=w7845) -> ("read buffer"=w7847:string)  [unwired: 10 in]
                                n7388 = call <vilib>:"Trim Whitespace.vi"("string"=w7847) -> ("trimmed string"=w7846:string)  [unwired: 1 in]
                                n7389 = Equal?(x=w7846, y="/0`\u0003") -> (x = y?=w7843:bool)
                                n7390 = Or(x=w7843, y=w7844) -> (x .or. y?=w7842:bool)
                                }
                                }
                              }
                            }
                            frame #9 {
                              n7391 = local read "Stop for End of \nExperiment \nand Data Writing"() -> (w7849:bool)
                              n7392 = local write "Pause Data Collection"(TRUE ("Pause Data Collection")) -> ()
                              n7393 = local write "Valve V2 Open"(FALSE ("Valve V2 Open")) -> ()
                              n7394 = local write "Valve V1 Open"(FALSE ("Valve V1 Open")) -> ()
                              n7395 = local write "Valve V3 Open"(FALSE ("Valve V3 Open")) -> ()
                              n7396 = local write "Valve V4 Open"(FALSE ("Valve V4 Open")) -> ()
                              n7397 = Wait (ms)(milliseconds to wait=u32 500) -> ()  [unwired: 1 out]
                              n7398 = case shown="True" w7849 {
                                frame False {
                                }
                                frame True {
                                n7399 = local read "VISA Refnum in\nfor Pump"() -> (w7859:refnum<visa-resource-name>)
                                n7400 = call "HardStopCurrentProcess (SubVI).vi"("VISA Refnum in"=w7859) -> ()  [unwired: 11 in]
                                }
                              }
                              n7401 = local write "Valve V6 Open"(FALSE ("Valve V6 Open")) -> ()
                              n7402 = local write "Valve V5 Open"(FALSE ("Valve V5 Open")) -> ()
                              n7403 = local write "Valve V7 Open"(FALSE ("Valve V7 Open")) -> ()
                            }
                            frame #10 {
                              n7404 = local write "Volume being Injected \nin this process"(0.0 ("Volume being Injected \nin this process")) -> ()
                            }
                          }
                        }
                        n7405 = local write "Reminder of the \nVolume to be \nPumped"(w7773) -> ()
                      }
                      frame #1 {
                        n7406 = stacked-sequence {
                          frame #0 {
                            # "Switch to Port-5/8"
                            # "Port-5/8 of pump is connected to Buffer-C/Buffer-A"
                            n7407 = local read "VISA Refnum in\nfor Pump"() -> (w7862:refnum<visa-resource-name>)
                            n7408 = local read "Port for \nC2-Elution"() -> (w7861:string)
                            n7409 = call "PortChanger (SubVI).vi"("Port Number"=w7861, "VISA Refnum in"=w7862) -> ()  [unwired: 10 in]
                          }
                          frame #1 {
                            n7410 = local read "VISA Refnum in\nfor Pump"() -> (w7863:refnum<visa-resource-name>)
                            n7411 = call "ProcessCompletionWaiter (SubVI).vi"("VISA Refnum in"=w7863) -> ()  [unwired: 11 in]
                          }
                          frame #2 {
                            n7412 = local read "Buffer-C2 PickUp \nFlow Rate (ul/min)"() -> (w7866:dbl)
                            n7413 = local read "Buffer-C2 Pumping\nResolution"() -> (w7865:T2)
                            n7414 = local read "VISA Refnum in\nfor Pump"() -> (w7868:refnum<visa-resource-name>)
                            n7415 = local read "Reminder of the \nVolume to be \nPumped"() -> (w7864:dbl)
                            n7416 = local read "Volume of Syringe"() -> (w7867:dbl)
                            n7417 = call "RPickUp(SubVI).vi"("Volume to be picked up"=w7864, "Volume of Syringe"=w7867, "Resolution of PickUP"=w7865, "PickUp Flow Rate (ul/min)"=w7866, "VISA Refnum in"=w7868) -> ()  [unwired: 6 in, 1 out]
                          }
                          frame #3 {
                            n7418 = local read "Stopper that ends \nthe main loops"() -> (w7869:bool)
                            n7419 = local read "VISA Refnum in\nfor Pump"() -> (w7870:refnum<visa-resource-name>)
                            n7420 = case shown="True" w7869 {
                              frame False {
                              }
                              frame True {
                                n7421 = local read "VISA Refnum in\nfor Pump"() -> (w7871:refnum<visa-resource-name>)
                                n7422 = call "HardStopCurrentProcess (SubVI).vi"("VISA Refnum in"=w7871) -> ()  [unwired: 11 in]
                              }
                            }
                            n7423 = call "ProcessCompletionWaiter (SubVI).vi"("VISA Refnum in"=w7870) -> ()  [unwired: 11 in]
                          }
                          frame #4 {
                            # "Reads the initial Plunger Position for computing the volume dispensed"
                            n7424 = local read "VISA Refnum in\nfor Pump"() -> (w7873:refnum<visa-resource-name>)
                            n7425 = call "AbsolutePlungerPosition (SubVI).vi"("VISA Refnum in"=w7873) -> ("Plunger Position"=w7872:i32)  [unwired: 10 in]
                            n7426 = local write "Initial Plunger Position"(w7872) -> ()
                          }
                          frame #5 {
                            # "Switch to Port-10"
                            # "Port-10 of the pump is conncted to column-2 of chip"
                            n7427 = local read "VISA Refnum in\nfor Pump"() -> (w7875:refnum<visa-resource-name>)
                            n7428 = call "PortChanger (SubVI).vi"("Port Number"="10", "VISA Refnum in"=w7875) -> ()  [unwired: 10 in]
                          }
                          frame #6 {
                            n7429 = local read "Stopper that ends \nthe main loops"() -> (w7876:bool)
                            n7430 = local read "VISA Refnum in\nfor Pump"() -> (w7877:refnum<visa-resource-name>)
                            n7431 = case shown="True" w7876 {
                              frame False {
                              }
                              frame True {
                                n7432 = local read "VISA Refnum in\nfor Pump"() -> (w7878:refnum<visa-resource-name>)
                                n7433 = call "HardStopCurrentProcess (SubVI).vi"("VISA Refnum in"=w7878) -> ()  [unwired: 11 in]
                              }
                            }
                            n7434 = call "ProcessCompletionWaiter (SubVI).vi"("VISA Refnum in"=w7877) -> ()  [unwired: 11 in]
                          }
                          frame #7 {
                            # "Keeps the AMF valve after column-1 closed and valve after column-2 open"
                            n7435 = local read "Buffer-C2 Dispense\nFlow Rate (ul/min)"() -> (w7891:dbl)
                            n7436 = local read "Buffer-C2 Pumping\nResolution"() -> (w7890:T2)
                            n7437 = local read "VISA Refnum in\nfor Pump"() -> (w7893:refnum<visa-resource-name>)
                            n7438 = local write "Pause Data Collection"(FALSE ("Pause Data Collection")) -> ()
                            n7439 = local write "Valve V1 Open"(FALSE ("Valve V1 Open")) -> ()
                            n7440 = local write "Valve V3 Open"(TRUE ("Valve V3 Open")) -> ()
                            n7441 = local write "Valve V2 Open"(FALSE ("Valve V2 Open")) -> ()
                            n7442 = local write "Valve V4 Open"(TRUE ("Valve V4 Open")) -> ()
                            n7443 = local read "Volume of Syringe"() -> (w7892:dbl)
                            n7444 = call "GoToAbsolutePosition(SubVI).vi"("Absolute Volume Position in Syringe (in ul)"=0.0 ("Volume to be Dispensed"), "Volume of Syringe"=w7892, "Resolution of Pumping"=w7890, "Flow Rate (ul/min)"=w7891, "VISA Refnum in"=w7893) -> ()  [unwired: 6 in, 1 out]
                            n7445 = local write "External Valve \nOpen"(FALSE ("External Valve \nOpen")) -> ()
                            n7446 = local write "Valve V8 Open"(FALSE ("Valve V8 Open")) -> ()
                            n7447 = local write "Valve V7 Open"(TRUE ("Valve V7 Open")) -> ()
                            n7448 = local write "Valve V6 Open"(TRUE ("Valve V6 Open")) -> ()
                            n7449 = local write "Valve V5 Open"(TRUE ("Valve V5 Open")) -> ()
                          }
                          frame #8 {
                            n7450 = local read "Initial Plunger Position"() -> (w7896:dbl)
                            n7451 = local read "Buffer-C2 Pumping\nResolution"() -> (w7895:T2)
                            n7452 = local read "VISA Refnum in\nfor Pump"() -> (w7897:refnum<visa-resource-name>)
                            n7453 = local read "Volume of Syringe"() -> (w7894:dbl)
                            n7454 = while {
                              tunnel: w7896 -> [w7903]
                              tunnel: w7897 -> [w7902]
                              tunnel: w7895 -> [w7901]
                              tunnel: w7894 -> [w7900]
                              stop <- w7898 stop-if-true
                              n7455 = Wait (ms)(milliseconds to wait=u32 100) -> ()  [unwired: 1 out]
                              n7456 = stacked-sequence {
                                tunnel: w7903 -> [w7909 _]
                                tunnel: w7902 -> [w7908 w7929]
                                tunnel: w7901 -> [w7907 _]
                                tunnel: w7900 -> [w7906 _]
                                tunnel: [_ w7926] -> w7898
                                frame #0 {
                                n7457 = call "AbsolutePlungerPosition (SubVI).vi"("VISA Refnum in"=w7908) -> ("Plunger Position"=w7905:i32)  [unwired: 10 in]
                                n7458 = case shown="\"Standard Pumping\", Default" w7907 {
                                tunnel: w7909 -> [w7914 w7923]
                                tunnel: w7905 -> [w7915 w7922]
                                tunnel: [w7913 w7920] -> w7904
                                tunnel: w7906 -> [w7912 w7921]
                                frame "Standard Pumping", Default {
                                n7459 = Subtract(x=w7914, y=w7915) -> (x-y=w7911:dbl)
                                n7460 = Absolute Value(x=w7911) -> (abs(x)=w7910:dbl)
                                n7461 = Multiply(x=w7910, y=w7912) -> (x*y=w7917:dbl)
                                n7462 = Divide(x=w7917, y=3000.0) -> (x/y=w7913:dbl)
                                }
                                frame "High Resolution Pumping" {
                                n7463 = Subtract(x=w7923, y=w7922) -> (x-y=w7919:dbl)
                                n7464 = Absolute Value(x=w7919) -> (abs(x)=w7918:dbl)
                                n7465 = Multiply(x=w7918, y=w7921) -> (x*y=w7925:dbl)
                                n7466 = Divide(x=w7925, y=24000.0) -> (x/y=w7920:dbl)
                                }
                                }
                                n7467 = local write "Volume being Injected \nin this process"(w7904) -> ()
                                }
                                frame #1 {
                                n7468 = call "LSPOneStatus (SubVI).vi"("VISA Refnum in"=w7929) -> ("read buffer"=w7931:string)  [unwired: 10 in]
                                n7469 = local read "Stopper that ends \nthe main loops"() -> (w7928:bool)
                                n7470 = call <vilib>:"Trim Whitespace.vi"("string"=w7931) -> ("trimmed string"=w7930:string)  [unwired: 1 in]
                                n7471 = Equal?(x=w7930, y="/0`\u0003") -> (x = y?=w7927:bool)
                                n7472 = Or(x=w7927, y=w7928) -> (x .or. y?=w7926:bool)
                                }
                              }
                            }
                          }
                          frame #9 {
                            n7473 = local read "Stop for End of \nExperiment \nand Data Writing"() -> (w7933:bool)
                            n7474 = local write "Pause Data Collection"(TRUE ("Pause Data Collection")) -> ()
                            n7475 = local write "Valve V2 Open"(FALSE ("Valve V2 Open")) -> ()
                            n7476 = local write "Valve V1 Open"(FALSE ("Valve V1 Open")) -> ()
                            n7477 = local write "Valve V3 Open"(FALSE ("Valve V3 Open")) -> ()
                            n7478 = local write "Valve V4 Open"(FALSE ("Valve V4 Open")) -> ()
                            n7479 = local write "Start the Process"(FALSE) -> ()
                            n7480 = Wait (ms)(milliseconds to wait=u32 500) -> ()  [unwired: 1 out]
                            n7481 = case shown="True" w7933 {
                              frame False {
                              }
                              frame True {
                                n7482 = local read "VISA Refnum in\nfor Pump"() -> (w7946:refnum<visa-resource-name>)
                                n7483 = call "HardStopCurrentProcess (SubVI).vi"("VISA Refnum in"=w7946) -> ()  [unwired: 11 in]
                              }
                            }
                            n7484 = local write "External Valve \nOpen"(FALSE ("External Valve \nOpen")) -> ()
                            n7485 = local write "Valve V8 Open"(FALSE ("Valve V8 Open")) -> ()
                            n7486 = local write "Valve V6 Open"(FALSE ("Valve V6 Open")) -> ()
                            n7487 = local write "Valve V5 Open"(FALSE ("Valve V5 Open")) -> ()
                            n7488 = local write "Valve V7 Open"(FALSE ("Valve V7 Open")) -> ()
                          }
                          frame #10 {
                            n7489 = local write "Volume being Injected \nin this process"(0.0 ("Volume being Injected \nin this process")) -> ()
                          }
                        }
                      }
                    }
                  }
                }
              }
              frame True {
                n7490 = local write "Pause Data Collection"(FALSE ("Pause Data Collection")) -> ()
              }
            }
          }
          frame "Initialize Only the Valve" {
            n7491 = local read "Stop for End of \nExperiment \nand Data Writing"() -> (w7949:bool)
            n7492 = case shown="False" w7949 {
              frame False {
                n7493 = local read "Start the Process"() -> (w7950:bool)
                n7494 = case shown="True" w7950 {
                  frame False {
                    n7495 = local read "Stopper that ends \nthe main loops"() -> (w7952:bool)
                    n7496 = local read "Start the Process"() -> (w7953:bool)
                    n7497 = Or(x=w7953, y=w7952) -> (x .or. y?=w7951:bool)
                    n7498 = case shown="False" w7951 {
                      frame False {
                        n7499 = while {
                          stop <- w7956 stop-if-true
                          n7500 = local read "Stopper that ends \nthe main loops"() -> (w7958:bool)
                          n7501 = local read "Start the Process"() -> (w7957:bool)
                          n7502 = Or(x=w7957, y=w7958) -> (x .or. y?=w7956:bool)
                          n7503 = Wait (ms)(milliseconds to wait=u32 10) -> ()  [unwired: 1 out]
                        }
                        n7504 = One Button Dialog(message="Please select the process and press the 'Start Process' Button") -> ()  [unwired: 1 in, 1 out]
                      }
                      frame True {
                      }
                    }
                  }
                  frame True {
                    n7505 = stacked-sequence {
                      frame #0 {
                        n7506 = local read "VISA Refnum in\nfor Valve"() -> (w7959:refnum<visa-resource-name>)
                        n7507 = call "Initializer_Valve (SubVI).vi"("VISA Refnum in"=w7959) -> ()  [unwired: 11 in]
                      }
                      frame #1 {
                        n7508 = local read "VISA Refnum in\nfor Valve"() -> (w7960:refnum<visa-resource-name>)
                        n7509 = call "ProcessCompletionWaiter (SubVI).vi"("VISA Refnum in"=w7960) -> ()  [unwired: 11 in]
                      }
                      frame #2 {
                        n7510 = local write "Start the Process"(FALSE ("Start the Process")) -> ()
                      }
                    }
                  }
                }
              }
              frame True {
              }
            }
          }
          frame "Clean the tubing from Ports 3,4,5 and 7" {
            n7511 = local read "Stopper that ends \nthe main loops"() -> (w7962:bool)
            n7512 = case shown="False" w7962 {
              frame False {
                n7513 = local read "Start the Process"() -> (w7963:bool)
                n7514 = case shown="True" w7963 {
                  frame False {
                    n7515 = local read "Stopper that ends \nthe main loops"() -> (w7965:bool)
                    n7516 = local read "Start the Process"() -> (w7964:bool)
                    n7517 = Or(x=w7965, y=w7964) -> (x .or. y?=w7966:bool)
                    n7518 = case shown="False" w7966 {
                      frame False {
                        n7519 = while {
                          stop <- w7969 stop-if-true
                          n7520 = local read "Stopper that ends \nthe main loops"() -> (w7971:bool)
                          n7521 = local read "Stop for End of \nExperiment \nand Data Writing"() -> (w7968:bool)
                          n7522 = local read "Start the Process"() -> (w7970:bool)
                          n7523 = Wait (ms)(milliseconds to wait=u32 10) -> ()  [unwired: 1 out]
                          n7524 = Or(x=w7971, y=w7970) -> (x .or. y?=w7969:bool)
                          n7525 = local write "Stopper that ends \nthe main loops"(w7968) -> ()
                        }
                        n7526 = One Button Dialog(message="Please Select the Process and Press 'Start the Process' Button") -> ()  [unwired: 1 in, 1 out]
                      }
                      frame True {
                      }
                    }
                  }
                  frame True {
                    n7527 = stacked-sequence {
                      frame #0 {
                        n7528 = for {
                          N: 2 -> [_]
                          n7529 = stacked-sequence {
                            frame #0 {
                              # "Switch to Port-4"
                              # "Port-4 of pump is connected to Buffer-A"
                              n7530 = local read "VISA Refnum in\nfor Pump"() -> (w7976:refnum<visa-resource-name>)
                              n7531 = local write "Pause Data Collection"(TRUE ("Pause Data Collection")) -> ()
                              n7532 = call "PortChanger (SubVI).vi"("Port Number"="3", "VISA Refnum in"=w7976) -> ()  [unwired: 10 in]
                            }
                            frame #1 {
                              n7533 = local read "VISA Refnum in\nfor Pump"() -> (w7977:refnum<visa-resource-name>)
                              n7534 = call "ProcessCompletionWaiter (SubVI).vi"("VISA Refnum in"=w7977) -> ()  [unwired: 11 in]
                            }
                            frame #2 {
                              n7535 = local read "VISA Refnum in\nfor Pump"() -> (w7982:refnum<visa-resource-name>)
                              n7536 = local read "Volume of Syringe"() -> (w7981:dbl)
                              n7537 = call "RPickUp(SubVI).vi"("Volume to be picked up"=10.0, "Volume of Syringe"=w7981, "Resolution of PickUP"=T2."Standard Pumping", "PickUp Flow Rate (ul/min)"=15.0, "VISA Refnum in"=w7982) -> ()  [unwired: 6 in, 1 out]
                            }
                            frame #3 {
                              n7538 = local read "Stopper that ends \nthe main loops"() -> (w7983:bool)
                              n7539 = local read "VISA Refnum in\nfor Pump"() -> (w7984:refnum<visa-resource-name>)
                              n7540 = case shown="True" w7983 {
                                frame False {
                                }
                                frame True {
                                n7541 = local read "VISA Refnum in\nfor Pump"() -> (w7985:refnum<visa-resource-name>)
